vi "Read XML_Extra Checks_Check BCD Parameters Bits Settings_Valid Combination.vi"(11 "Parameter":T1) -> (3 "Not Valid":bool)   [LabVIEW 2016]
uses:
  XML_Parameter.ctl
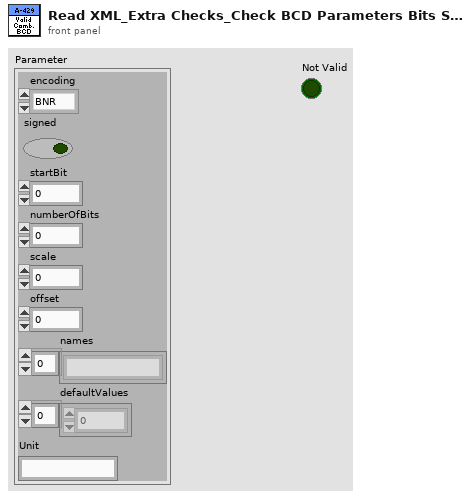
[diagram p1: front panel]
types:
  T1 = typedef "XML_Parameter.ctl" = cluster{"encoding":enum16{"BNR", "BCD", "Discrete"}, "signed":bool, "startBit":i32, "numberOfBits":i32, "scale":dbl, "offset":dbl, "names":string[], "defaultValues":dbl[], "Unit":string}
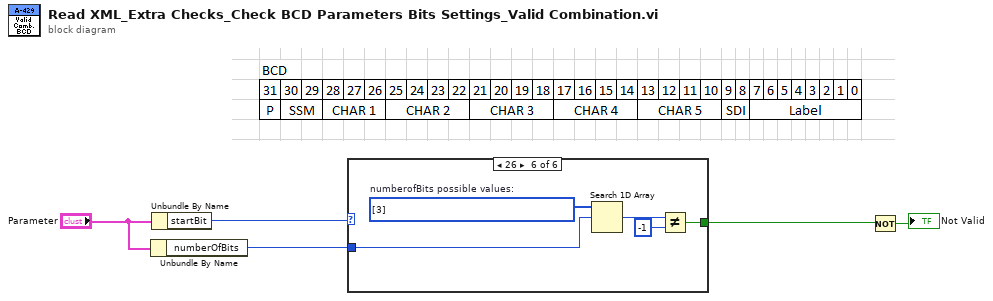
[diagram p0: block diagram]
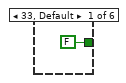
[diagram p2: hidden frame]
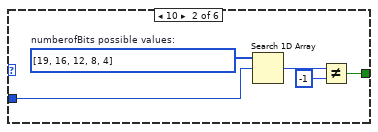
[diagram p3: hidden frame]
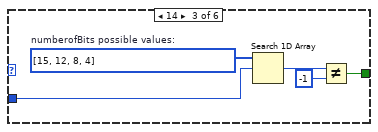
[diagram p4: hidden frame]
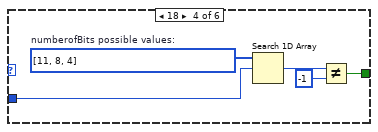
[diagram p5: hidden frame]
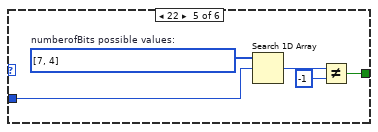
[diagram p6: hidden frame]
diagram:
  n1 = Unbundle By Name("Parameter") -> ("numberOfBits"=w2:i32)
  n2 = Unbundle By Name("Parameter") -> ("startBit"=w3:i32)
  n3 = case shown="26" w3 {
    tunnel: w2 -> [_ w8 w13 w18 w23 w28]
    tunnel: [FALSE w7 w12 w17 w22 w27] -> w1
    frame 33, Default {
    }
    frame 10 {
      w9 = i32[] [19, 16, 12, 8, 4]  # numberofBits possible values:
      n4 = Search 1D Array(1D array=w9, element=w8) -> (index of element=w10:i32)  [unwired: 1 in]
      n5 = Not Equal?(x=w10, y=-1) -> (x != y?=w7:bool)
    }
    frame 14 {
      w14 = i32[] [15, 12, 8, 4]  # numberofBits possible values:
      n6 = Search 1D Array(1D array=w14, element=w13) -> (index of element=w15:i32)  [unwired: 1 in]
      n7 = Not Equal?(x=w15, y=-1) -> (x != y?=w12:bool)
    }
    frame 18 {
      w19 = i32[] [11, 8, 4]  # numberofBits possible values:
      n8 = Search 1D Array(1D array=w19, element=w18) -> (index of element=w20:i32)  [unwired: 1 in]
      n9 = Not Equal?(x=w20, y=-1) -> (x != y?=w17:bool)
    }
    frame 22 {
      w24 = i32[] [7, 4]  # numberofBits possible values:
      n10 = Search 1D Array(1D array=w24, element=w23) -> (index of element=w25:i32)  [unwired: 1 in]
      n11 = Not Equal?(x=w25, y=-1) -> (x != y?=w22:bool)
    }
    frame 26 {
      w29 = i32[] [3]  # numberofBits possible values:
      n12 = Search 1D Array(1D array=w29, element=w28) -> (index of element=w30:i32)  [unwired: 1 in]
      n13 = Not Equal?(x=w30, y=-1) -> (x != y?=w27:bool)
    }
  }
  n14 = Not(x=w1) -> (.not. x?=→"Not Valid":bool)
